vi "high_pass_filter_1st.vi"(7 "Input":dbl format="%.2f", 13 "Corner period":dbl(slide)=10.237739663395852 scale=1.0..1000.0) -> (8 "Output":dbl format="%.2f")   [LabVIEW 2016]
doc: "Use this VI to filter a signal using 1st order high pass filter. The difference equation is\nv0(j) =[ Vo(j-1) + Vi(j) - Vi(j-1)] / [b + 1].\n\nInputs:\nInput,\nCorner period.\nOutputs:\nOutput.\n\nMuhannad Alghamdi\nCSUSB Physics 350"
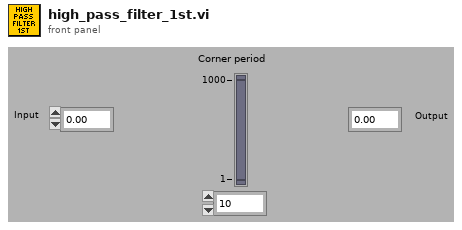
[diagram p1: front panel]
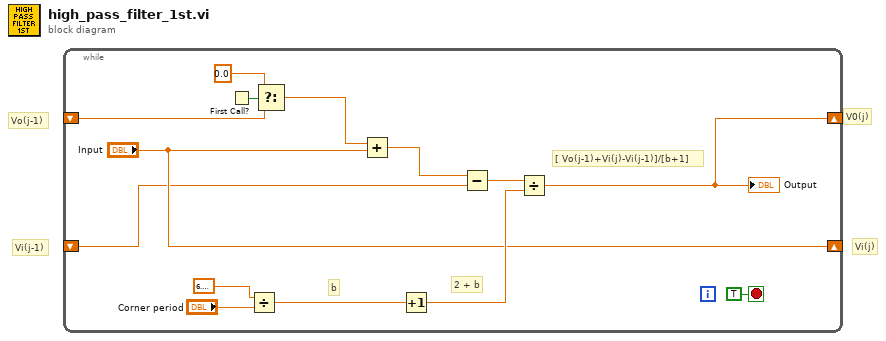
[diagram p0: block diagram]
diagram:
  # "Vi(j-1)"
  # "Vo(j-1)"
  # "Vi(j)"
  # "V0(j)"
  n1 = while {
    shift-left: _ -> [w7]
    shift-right: [w9] -> _
    shift-right: ["Input"] -> _
    shift-left: _ -> [w1]
    stop <- TRUE stop-if-true
    # "[ Vo(j-1)+Vi(j)-Vi(j-1)]/[b+1]"
    # "b"
    # "2 + b"
    n2 = First Call?() -> (First Call?: T/F=w8:bool)
    n3 = Divide(x=6.283185307179586, y="Corner period") -> (x/y=w11:dbl)
    n4 = Select(t=0.0, s=w8, f=w7) -> (s? t:f=w6:dbl)
    n5 = Add(x=w6, y="Input") -> (x+y=w4:dbl)
    n6 = Increment(x=w11) -> (x+1=w10:dbl)
    n7 = Subtract(x=w4, y=w1) -> (x-y=w3:dbl)
    n8 = Divide(x=w3, y=w10) -> (x/y=w9:dbl)
    "Output" <- w9
  }
